vi "startBoard.vi"() -> ()   [LabVIEW 2020]
panel:
  out "output array":i32[][](array[numeric])
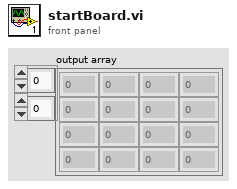
[diagram p1: front panel]
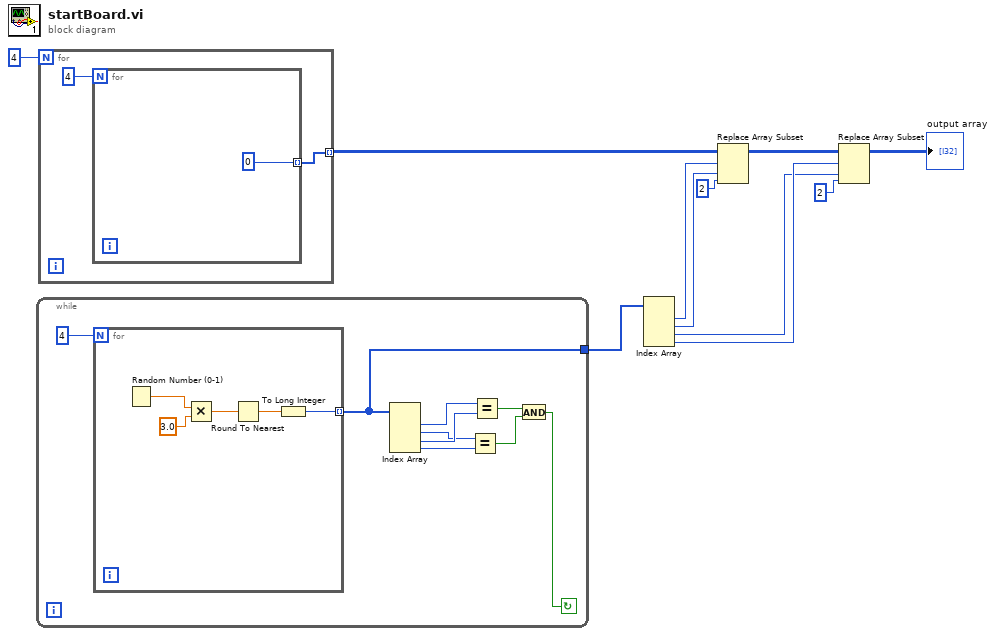
[diagram p0: block diagram]
diagram:
  n1 = while {
    tunnel: [w13] -> w10
    stop <- w12 continue-if-true
    n2 = for {
      N: 4 -> [_]
      tunnel: [w22] -> w13 mode=indexing
      n3 = Random Number (0-1)() -> (number: 0 to 1=w25:dbl)
      n4 = Multiply(x=w25, y=3.0) -> (x*y=w24:dbl)
      n5 = Round To Nearest(number=w24) -> (nearest integer value=w23:dbl)
      n6 = To Long Integer(number=w23) -> (32bit integer=w22:i32)
    }
    n7 = Index Array(array=w13) -> (element #1=w19:i32, element #2=w17:i32, element #3=w18:i32, element #4=w16:i32)  [unwired: 4 in]
    n8 = Equal?(x=w17, y=w16) -> (x = y?=w14:bool)
    n9 = Equal?(x=w19, y=w18) -> (x = y?=w15:bool)
    n10 = And(x=w15, y=w14) -> (x .and. y?=w12:bool)
  }
  n11 = for {
    N: 4 -> [_]
    tunnel: [w26] -> w9 mode=indexing
    n12 = for {
      N: 4 -> [_]
      tunnel: [0] -> w26 mode=indexing
    }
  }
  n13 = Index Array(array=w10) -> (element #1=w2:i32, element #2=w1:i32, element #3=w3:i32, element #4=w4:i32)  [unwired: 4 in]
  n14 = Replace Array Subset(array=w9, new element=2, index (row)=w2, index (col)=w1) -> (w8:i32[][])
  n15 = Replace Array Subset(array=w8, new element=2, index (row)=w4, index (col)=w3) -> (→"output array":i32[][])
